vi "Node Style to ID.vi"(11 "Function Name":string) -> (2 "key not found?":bool, 3 "Function ID":i32)   [LabVIEW 2020]
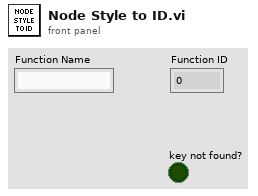
[diagram p1: front panel]
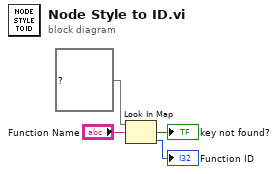
[diagram p0: block diagram]
diagram:
  n1 = Look In Map(map=map{string, i32} data[31583B] ("map in"), key="Function Name") -> (key not found?=→"key not found?":bool, value=→"Function ID":i32)  [unwired: 1 in]
